vi "1-2.vi"() -> ()   [LabVIEW 2022 SP3]
panel:
  out "数值 3":dbl
  out "数值 2":dbl
  out "数值":dbl
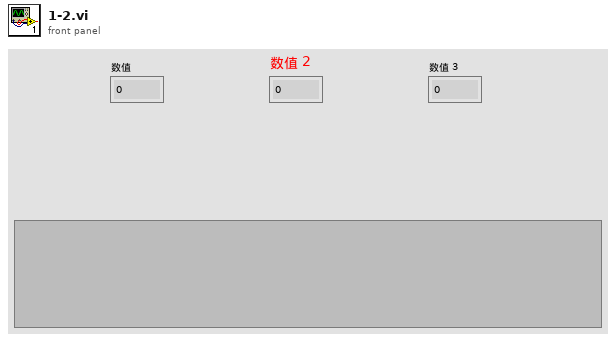
[diagram p1: front panel]
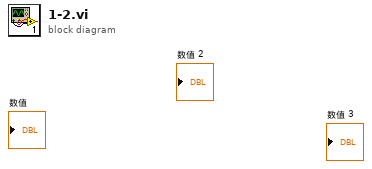
[diagram p0: block diagram]
diagram:
